vi "HFRR ADV v022 new software.vi"() -> ()   [LabVIEW 2025] (continued)
            n2951 = Match Pattern(string=w3831, regular expression=".dgf" ("substring (\"\")")) -> (before substring=w3841:string)  [unwired: 1 in, 3 out]
            n2952 = Concatenate Strings(w3841, ".duf" ("Substring")) -> (w3837:string)
            n2953 = String To Path(string=w3837) -> (path=w3842:path)
            n2954 = call <vilib>:"Read Characters From File.vi"("file path (dialog if empty)"=w3842, "start of read offset (chars.:0)"=60 ("start of read offset (chars.: 0)")) -> ("character string"=→"String Control 2":string)  [unwired: 4 in, 3 out]
          }
        }
        n2955 = case shown="True" "OPEN 2" {
          frame False {
          }
          frame True {
            (unwired) 0  # existing file
            w3863 = "Choose a datalog file to open"  # prompt
            n2956 = local write "OPEN 2"(FALSE ("OPEN 1")) -> ()
            n2957 = String To Path(string="C:\\LAB-IQ\\Data\\") -> (path=w3848:path)
            n2958 = File Dialog(6:"*.dgf" ("pattern"), 7:w3863, 11:w3848) -> (0:w3846:errorcluster, 3:w3854:path)  [unwired: 4 in, 2 out]
            n2959 = Unbundle(w3846) -> ()  [unwired: 3 out]
            n2960 = Strip Path(path=w3854) -> (name=w3852:string)  [unwired: 1 out]
            n2961 = Path To String(path=w3854) -> (string=w3849:string)
            "string1 2" <- w3849
            n2962 = Match Pattern(string=w3852, regular expression=".dgf") -> (before substring=→"String Control 3":string)  [unwired: 1 in, 3 out]
            n2963 = Match Pattern(string=w3849, regular expression=".dgf" ("substring (\"\")")) -> (before substring=w3860:string)  [unwired: 1 in, 3 out]
            n2964 = Concatenate Strings(w3860, ".duf" ("Substring")) -> (w3857:string)
            n2965 = String To Path(string=w3857) -> (path=w3855:path)
            n2966 = call <vilib>:"Read Characters From File.vi"("file path (dialog if empty)"=w3855, "start of read offset (chars.:0)"=60 ("start of read offset (chars.: 0)")) -> ("character string"=→"String Control 4":string)  [unwired: 4 in, 3 out]
          }
        }
        n2967 = case shown="True" "OPEN 3" {
          frame False {
          }
          frame True {
            (unwired) 0  # existing file
            w3881 = "Choose a datalog file to open"  # prompt
            n2968 = local write "OPEN 3"(FALSE ("OPEN 1")) -> ()
            n2969 = String To Path(string="C:\\LAB-IQ\\Data\\") -> (path=w3866:path)
            n2970 = File Dialog(6:"*.dgf" ("pattern"), 7:w3881, 11:w3866) -> (0:w3864:errorcluster, 3:w3872:path)  [unwired: 4 in, 2 out]
            n2971 = Unbundle(w3864) -> ()  [unwired: 3 out]
            n2972 = Strip Path(path=w3872) -> (name=w3870:string)  [unwired: 1 out]
            n2973 = Path To String(path=w3872) -> (string=w3867:string)
            "string1 3" <- w3867
            n2974 = Match Pattern(string=w3870, regular expression=".dgf") -> (before substring=→"String Control 5":string)  [unwired: 1 in, 3 out]
            n2975 = Match Pattern(string=w3867, regular expression=".dgf" ("substring (\"\")")) -> (before substring=w3877:string)  [unwired: 1 in, 3 out]
            n2976 = Concatenate Strings(w3877, ".duf" ("Substring")) -> (w3874:string)
            n2977 = String To Path(string=w3874) -> (path=w3878:path)
            n2978 = call <vilib>:"Read Characters From File.vi"("file path (dialog if empty)"=w3878, "start of read offset (chars.:0)"=60 ("start of read offset (chars.: 0)")) -> ("character string"=→"String Control 6":string)  [unwired: 4 in, 3 out]
          }
        }
        n2979 = case shown="True" "OPEN 4" {
          frame False {
          }
          frame True {
            (unwired) 0  # existing file
            w3899 = "Choose a datalog file to open"  # prompt
            n2980 = local write "OPEN 4"(FALSE ("OPEN 1")) -> ()
            n2981 = String To Path(string="C:\\LAB-IQ\\Data\\") -> (path=w3884:path)
            n2982 = File Dialog(6:"*.dgf" ("pattern"), 7:w3899, 11:w3884) -> (0:w3882:errorcluster, 3:w3890:path)  [unwired: 4 in, 2 out]
            n2983 = Unbundle(w3882) -> ()  [unwired: 3 out]
            n2984 = Strip Path(path=w3890) -> (name=w3888:string)  [unwired: 1 out]
            n2985 = Path To String(path=w3890) -> (string=w3885:string)
            "string1 4" <- w3885
            n2986 = Match Pattern(string=w3888, regular expression=".dgf") -> (before substring=→"String Control 7":string)  [unwired: 1 in, 3 out]
            n2987 = Match Pattern(string=w3885, regular expression=".dgf" ("substring (\"\")")) -> (before substring=w3895:string)  [unwired: 1 in, 3 out]
            n2988 = Concatenate Strings(w3895, ".duf" ("Substring")) -> (w3892:string)
            n2989 = String To Path(string=w3892) -> (path=w3896:path)
            n2990 = call <vilib>:"Read Characters From File.vi"("file path (dialog if empty)"=w3896, "start of read offset (chars.:0)"=60 ("start of read offset (chars.: 0)")) -> ("character string"=→"String Control 8":string)  [unwired: 4 in, 3 out]
          }
        }
      }
      frame "About" {
        # "Elapsed time\ncof\nstroke\nmean pos\nTemp\nHumidity"
        n2991 = disable-structure shown="Disabled" {
          frame Disabled {
            n2992 = case shown="True" "Export" {
              frame False {
              }
              frame True {
                w3921 = "                                      " ("string")
                w3923 = "\r"
                (unwired) i16 6 ("width (-)")
                w4000 = "\r"
                w3932 = "\r"
                n2993 = local write "Export"(FALSE ("Export")) -> ()
                n2994 = local read "String 29"() -> (w3969:string)
                n2995 = local read "String 34"() -> (w3957:string)
                n2996 = local read "String 35"() -> (w3952:string)
                n2997 = local read "String 37"() -> (w3948:string)
                n2998 = local read "String 36"() -> (w3945:string)
                n2999 = local read "String 38"() -> (w3942:string)
                n3000 = local read "String 39"() -> (w3939:string)
                n3001 = Match Pattern(string=w3969, regular expression=".dwm") -> (before substring=w3965:string)  [unwired: 1 in, 3 out]
                "before substring" <- w3965
                n3002 = local read "S 38"() -> (w3960:string)
                n3003 = local read "S 39"() -> (w3953:string)
                n3004 = local read "Temperature before test 2"() -> (w3989:dbl)
                n3005 = local read "Temperature after test 2"() -> (w3994:dbl)
                n3006 = local read "Humidity before test 2"() -> (w3975:dbl)
                n3007 = local read "Humidity after test 2"() -> (w3990:dbl)
                n3008 = local read "MWSD 2"() -> (w3986:dbl)
                n3009 = local read "WS1.4 2"() -> (w4002:dbl)
                n3010 = local read "HCF 2"() -> (w3998:dbl)
                n3011 = local read "AVP 2"() -> (w3987:dbl)
                n3012 = Concatenate Strings("1," ("string"), w3960) -> (w3959:string)
                n3013 = Concatenate Strings("2," ("string"), w3957) -> (w3956:string)
                n3014 = Concatenate Strings("3," ("string"), w3953) -> (w3955:string)
                n3015 = Concatenate Strings("4," ("string"), w3952) -> (w3951:string)
                n3016 = Concatenate Strings("5," ("string"), w3948) -> (w3949:string)
                n3017 = Concatenate Strings("6," ("string"), w3945) -> (w3946:string)
                n3018 = Concatenate Strings("7," ("string"), w3942) -> (w3943:string)
                n3019 = Concatenate Strings("8," ("string"), w3939) -> (w3940:string)
                n3020 = local read "Sample ID"() -> (w4007:string)
                n3021 = case shown="\"xlx\"" "Select File Type" {
                  tunnel: w3965 -> [w4010 w4012 w4014]
                  tunnel: [w4008 w4013 w4015] -> w3964
                  frame "xlx" {
                    n3022 = Concatenate Strings(w4010, ".xls" ("string")) -> (w4008:string)
                  }
                  frame "csv" {
                    n3023 = Concatenate Strings(w4012, ".csv" ("string")) -> (w4013:string)
                  }
                  frame "txt" {
                    n3024 = Concatenate Strings(w4014, ".txt" ("string")) -> (w4015:string)
                  }
                }
                n3025 = local read "Test Date"() -> (w4006:string)
                n3026 = local read "String 45"() -> (w3920:string)
                n3027 = local read "String 31"() -> (w4005:string)
                n3028 = local read "String 32"() -> (w4004:string)
                n3029 = local read "TITTLE"() -> (w3928:string)
                n3030 = Number To Fractional String(number=w3975, width (-)=i16 6, precision (6)=i16 2) -> (F-format string=w3974:string)  [unwired: 1 in]
                n3031 = Number To Fractional String(number=w3989, width (-)=i16 6, precision (6)=i16 2) -> (F-format string=w3995:string)  [unwired: 1 in]
                n3032 = Number To Fractional String(number=w3990, width (-)=i16 6, precision (6)=i16 2) -> (F-format string=w3988:string)  [unwired: 1 in]
                n3033 = Number To Fractional String(number=w3994, width (-)=i16 6, precision (6)=i16 2) -> (F-format string=w3993:string)  [unwired: 1 in]
                n3034 = Number To Fractional String(number=w3986, width (-)=i16 6, precision (6)=i16 2) -> (F-format string=w3984:string)  [unwired: 1 in]
                n3035 = Number To Fractional String(number=w3987, width (-)=i16 6, precision (6)=i16 2) -> (F-format string=w3985:string)  [unwired: 1 in]
                n3036 = Number To Fractional String(number=w3998, width (-)=i16 6, precision (6)=i16 2) -> (F-format string=w3999:string)  [unwired: 1 in]
                n3037 = Number To Fractional String(number=w4002, precision (6)=i16 2) -> (F-format string=w4003:string)  [unwired: 2 in]
                n3038 = local read "s.NO"() -> (w3922:string)
                n3039 = Concatenate Strings("=" ("string"), w3928) -> (w3927:string)
                n3040 = Concatenate Strings("S.No," ("string"), "                                       Parameters" ("string")) -> (w3933:string)
                n3041 = Concatenate Strings(w4000, w3959, w3974, w4000, w3956, w3995, w4000, w3955, w3988, w4000, w3951, w3993, w4000, w3949, w3984, w4000, w3946, w3985, w4000, w3943, w3999, w4000, w3940, w4003) -> (w3962:string)
                n3042 = Concatenate Strings(w3932, "," ("string"), w3920, w3922, w3921, w4004, w4007, w3921, w4005, w4006, w3932) -> (w3930:string)
                n3043 = local read "Tested by"() -> (w3936:string)
                n3044 = local read "String 33"() -> (w3937:string)
                n3045 = Concatenate Strings("," ("string"), "                                                                             " ("string")) -> (w3925:string)
                n3046 = Concatenate Strings(w3927, w3923, w3930, w3923, w3933, w3962, w3923, w3925, w3937, w3936) -> (→"export":string)
                n3047 = String To Path(string=w3964) -> (path=w3971:path)
                n3048 = local read "export"() -> (w3966:string)
                n3049 = call <vilib>:"Write Characters To File.vi"("append to file? (new file:F)"=FALSE, "character string"=w3966, "file path (dialog if empty)"=w3971) -> ()  [unwired: 2 in, 1 out]
              }
            }
          }
          frame Enabled {
          }
        }
        n3050 = case shown="True" "OK Button 17" {
          frame False {
          }
          frame True {
            (unwired) 0  # existing file
            w4224 = "Choose a datalog file to open"  # prompt
            n3051 = local write "OK Button 17"(FALSE ("OK Button 17")) -> ()
            n3052 = local read "String"() -> (w4219:string)
            n3053 = String To Path(string=w4219) -> (path=w4220:path)
            n3054 = File Dialog(6:"*.duf" ("pattern"), 7:w4224, 11:w4220) -> (0:w4211:errorcluster, 3:w4230:path)  [unwired: 4 in, 2 out]
            n3055 = Unbundle(w4211) -> ()  [unwired: 3 out]
            n3056 = Open/Create/Replace File "Open File"(file path (use dialog)=w4230) -> (refnum out=w4222:refnum<file>)  [unwired: 5 in, 2 out]
            n3057 = Strip Path(path=w4230) -> (name=w4228:string)  [unwired: 1 out]
            n3058 = Path To String(path=w4230) -> (string=w4213:string)
            n3059 = while {
              tunnel: w4222 -> [w4234]
              i -> [w4231]
              stop <- w4232 continue-if-true
              (unwired) TRUE ("line mode (F)")
              n3060 = Read from Text File "Read File"(file (use dialog)=w4234) -> (text=w4233:string)  [unwired: 3 in, 3 out]
              n3061 = local write "Numeric 16"(w4231) -> ()
              n3062 = String Length(string=w4233) -> (length=w4236:i32)
              n3063 = Greater?(x=w4236, y=1) -> (0:w4232:bool)
            }
            n3064 = local write "String 29"(w4213) -> ()
            n3065 = Search and Replace String(input string=w4213, search string=".duf", replace string=".dgf" ("replace string (\"\")")) -> (result string=→"String Indicator 4":string)  [unwired: 5 in, 3 out]
            n3066 = Match Pattern(string=w4228, regular expression=".dwm") -> (before substring=w4212:string)  [unwired: 1 in, 3 out]
            "String Indicator" <- w4212
            n3067 = Match Pattern(string=w4213, regular expression=".dwm" ("substring (\"\")")) -> (before substring=w4214:string)  [unwired: 1 in, 3 out]
            "String Indicator 3" <- w4214
            n3068 = local write "TITTLE 2"(w4212) -> ()
            n3069 = String To Path(string=w4214) -> (path=w4221:path)
            "path" <- w4221
            n3070 = call <vilib>:"Read Characters From File.vi"("file path (dialog if empty)"=w4221, "start of read offset (chars.:0)"=60 ("start of read offset (chars.: 0)")) -> ("character string"=→"String Indicator 2":string)  [unwired: 4 in, 3 out]
          }
        }
        n3071 = call <vilib>:"Query Available Printers.vi"() -> ("system configured printers"=w3913:string[])  [unwired: 9 in, 2 out]
        "System Configured Printers 2" <- w3913
        n3072 = local read "OK Button 16"() -> (w3910:bool)
        n3073 = case shown="True" "OK Button 16" {
          frame False {
          }
          frame True {
            n3074 = stacked-sequence {
              frame #0 {
                n3075 = local read "Numeric 16"() -> (w4238:i32)
                n3076 = local write "Numeric 10"(w4238) -> ()
              }
              frame #1 {
                n3077 = local read "S.NO"() -> (→"s.NO":string)
                n3078 = local read "String 29"() -> (w4242:string)
                n3079 = String To Path(string=w4242) -> (path=w4241:path)
                n3080 = Open/Create/Replace File "Open File"(file path (use dialog)=w4241) -> (refnum out=w4243:refnum<file>)  [unwired: 5 in, 2 out]
                n3081 = for {
                  N: 16 -> [_]
                  tunnel: w4243 -> [w4250]
                  i -> [w4246]
                  (unwired) TRUE ("line mode (F)")
                  n3082 = Read from Text File "Read File"(file (use dialog)=w4250) -> (text=w4244:string)  [unwired: 3 in, 3 out]
                  n3083 = Match Pattern(string=w4244, regular expression="(") -> (after substring=w4249:string)  [unwired: 1 in, 3 out]
                  n3084 = Match Pattern(string=w4249, regular expression=")") -> (before substring=w4245:string)  [unwired: 1 in, 3 out]
                  n3085 = case shown="1" w4246 {
                    tunnel: w4245 -> [w4251 w4252 _ _ w4253 w4254 w4255 w4257 w4259 w4261 w4263 w4265 w4267 w4269 _]
                    tunnel: w4244 -> [_ _ _ _ _ _ _ _ _ _ _ _ _ _ _]
                    frame 0 {
                      "TITTLE" <- w4251
                    }
                    frame 1 {
                      "Sample ID" <- w4252
                    }
                    frame 2 {
                    }
                    frame 3 {
                    }
                    frame 4 {
                      "Test Date" <- w4253
                    }
                    frame 5 {
                      "Tested by" <- w4254
                    }
                    frame 6 {
                      n3086 = Fract/Exp String To Number(string=w4255) -> (number=→"Humidity before test 2":dbl)  [unwired: 3 in, 1 out]
                    }
                    frame 7 {
                      n3087 = Fract/Exp String To Number(string=w4257) -> (number=→"Temperature before test 2":dbl)  [unwired: 3 in, 1 out]
                    }
                    frame 8 {
                      n3088 = Fract/Exp String To Number(string=w4259) -> (number=→"Humidity after test 2":dbl)  [unwired: 3 in, 1 out]
                    }
                    frame 9 {
                      n3089 = Fract/Exp String To Number(string=w4261) -> (number=→"Temperature after test 2":dbl)  [unwired: 3 in, 1 out]
                    }
                    frame 10 {
                      n3090 = Fract/Exp String To Number(string=w4263) -> (number=→"MWSD 2":dbl)  [unwired: 3 in, 1 out]
                    }
                    frame 11 {
                      n3091 = Fract/Exp String To Number(string=w4265) -> (number=→"AVP 2":dbl)  [unwired: 3 in, 1 out]
                    }
                    frame 12 {
                      n3092 = Fract/Exp String To Number(string=w4267) -> (number=→"HCF 2":dbl)  [unwired: 3 in, 1 out]
                    }
                    frame 13 {
                      n3093 = Fract/Exp String To Number(string=w4269) -> (number=→"WS1.4 2":dbl)  [unwired: 3 in, 1 out]
                    }
                    frame 14, Default {
                    }
                  }
                }
              }
              frame #2 {
              }
            }
            n3094 = local write "OK Button 16"(FALSE ("OK Button 13")) -> ()
          }
        }
        n3095 = Index Array(array=w3913, index="Select Printer 3") -> (element=w3915:string)
        "Selected Printer" <- w3915
        n3096 = case shown="True" w3910 {
          frame False {
          }
          frame True {
            n3097 = flat-sequence {
              frame #0 {
              }
              frame #1 {
                n3098 = Wait (ms)(milliseconds to wait=u32 100) -> ()  [unwired: 1 out]
              }
              frame #2 {
                n3099 = local write "OK Button 16"(FALSE ("Print 3")) -> ()
              }
            }
          }
        }
        n3100 = case shown="True" "Print" {
          tunnel: w3915 -> [_ w4207]
          frame False {
          }
          frame True {
            (unwired) i16 6 ("width (-)")
            (unwired) "TESTED BY : "
            (unwired) "TESTED DATE :"
            (unwired) "SAMPLE ID : "
            (unwired) "SAMPLE DESIGN : "
            w4165 = "\r"
            w4182 = "\r"
            # "add image"
            n3101 = local read "Sample ID"() -> (w4155:string)
            n3102 = local read "Tested by"() -> (w4158:string)
            n3103 = local read "String 34"() -> (w4145:string)
            n3104 = local read "String 45"() -> (w4125:string)
            n3105 = local read "String 35"() -> (w4140:string)
            n3106 = local read "String 37"() -> (w4138:string)
            n3107 = local read "String 32"() -> (w4160:string)
            n3108 = local read "String 36"() -> (w4135:string)
            n3109 = local read "String 31"() -> (w4159:string)
            n3110 = local read "Test Date"() -> (w4156:string)
            n3111 = local read "String 33"() -> (w4161:string)
            n3112 = local read "String 38"() -> (w4131:string)
            n3113 = local read "String 39"() -> (w4128:string)
            n3114 = local write "Print"(FALSE ("Print FF")) -> ()
            n3115 = local read "S 39"() -> (w4143:string)
            n3116 = local read "S 38"() -> (w4150:string)
            n3117 = local read "Temperature before test 2"() -> (w4181:dbl)
            n3118 = local read "Temperature after test 2"() -> (w4171:dbl)
            n3119 = local read "Humidity before test 2"() -> (w4196:dbl)
            n3120 = local read "Humidity after test 2"() -> (w4180:dbl)
            n3121 = local read "MWSD 2"() -> (w4185:dbl)
            n3122 = local read "WS1.4 2"() -> (w4163:dbl)
            n3123 = Concatenate Strings("2)" ("string"), w4145) -> (w4146:string)
            n3124 = Concatenate Strings("3)" ("string"), w4143) -> (w4144:string)
            n3125 = Concatenate Strings("1)" ("string"), w4150) -> (w4149:string)
            n3126 = Concatenate Strings("4)" ("string"), w4140) -> (w4141:string)
            n3127 = Concatenate Strings("5)" ("string"), w4138) -> (w4137:string)
            n3128 = Concatenate Strings("6)" ("string"), w4135) -> (w4134:string)
            n3129 = Concatenate Strings("7)" ("string"), w4131) -> (w4132:string)
            n3130 = Concatenate Strings("8)" ("string"), w4128) -> (w4129:string)
            n3131 = local read "HCF 2"() -> (w4167:dbl)
            n3132 = local read "AVP 2"() -> (w4184:dbl)
            n3133 = local read "s.NO"() -> (w4126:string)
            n3134 = call <vilib>:"New Report.vi"("report type"=enum16{"Standard Report", "HTML"}."Standard Report") -> ("report out"=w4205:refnum<class "NI_report.lvclass">, "error out"=w4204:errorcluster)  [unwired: 13 in]
            n3135 = local read "TITTLE"() -> (w4157:string)
            n3136 = Concatenate Strings(w4182, w4125, w4126, w4182, w4160, w4155, w4182, w4159, w4156, w4182, w4161, w4158, w4182) -> (w4175:string)
            "test by" <- w4175
            n3137 = Number To Fractional String(number=w4181, width (-)=i16 6, precision (6)=i16 2) -> (F-format string=w4170:string)  [unwired: 1 in]
            n3138 = Number To Fractional String(number=w4180, width (-)=i16 6, precision (6)=i16 2) -> (F-format string=w4183:string)  [unwired: 1 in]
            n3139 = Number To Fractional String(number=w4196, width (-)=i16 6, precision (6)=i16 2) -> (F-format string=w4201:string)  [unwired: 1 in]
            n3140 = Number To Fractional String(number=w4185, width (-)=i16 6, precision (6)=i16 2) -> (F-format string=w4187:string)  [unwired: 1 in]
            n3141 = Number To Fractional String(number=w4171, width (-)=i16 6, precision (6)=i16 2) -> (F-format string=w4172:string)  [unwired: 1 in]
            n3142 = Number To Fractional String(number=w4184, width (-)=i16 6, precision (6)=i16 2) -> (F-format string=w4186:string)  [unwired: 1 in]
            n3143 = Number To Fractional String(number=w4167, width (-)=i16 6, precision (6)=i16 2) -> (F-format string=w4166:string)  [unwired: 1 in]
            n3144 = Number To Fractional String(number=w4163, precision (6)=i16 2) -> (F-format string=w4162:string)  [unwired: 2 in]
            n3145 = call-dynamic "Set Report Header Text.vi"("report in"=w4205, "center header text"=w4157, "error in (no error)"=w4204) -> ("report out"=w4176:refnum<class "NI_report.lvclass">, "error out"=w4177:errorcluster)  [unwired: 11 in]
            n3146 = Concatenate Strings(w4165, w4149, w4201, w4165, w4146, w4170, w4165, w4144, w4183, w4165, w4141, w4172, w4165, w4137, w4187, w4165, w4134, w4186, w4165, w4132, w4166, w4165, w4129, w4162) -> (w4153:string)
            "export 2" <- w4153
            n3147 = call-poly <vilib>:"Append Report Text.vi"("report in"=w4176, "text"=w4175, "error in (no error)"=w4177) -> ("report out"=w4179:refnum<class "NI_report.lvclass">, "error out"=w4178:errorcluster)  [unwired: 9 in, 2 out]
            n3148 = local read "test by"() -> (w4152:string)
            n3149 = local read "TITTLE"() -> (w4154:string)
            n3150 = call-poly <vilib>:"Append Report Text.vi"("report in"=w4179, "error in (no error)"=w4178) -> ("report out"=w4200:refnum<class "NI_report.lvclass">, "error out"=w4198:errorcluster)  [unwired: 10 in, 2 out]
            n3151 = Concatenate Strings(w4154, w4153, w4152) -> (→"output":string)
            n3152 = call-poly <vilib>:"Append Report Text.vi"("report in"=w4200, "text"=w4153, "error in (no error)"=w4198) -> ("report out"=w4199:refnum<class "NI_report.lvclass">, "error out"=w4197:errorcluster)  [unwired: 9 in, 2 out]
            n3153 = call-dynamic "Print Report.vi"("report in"=w4199, "printer name (default)"=w4207, "error in (no error)"=w4197) -> ("report out"=w4209:refnum<class "NI_report.lvclass">, "error out"=w4210:errorcluster)  [unwired: 11 in]
            n3154 = call-dynamic "Dispose Report.vi"("report in"=w4209, "error in (no error)"=w4210) -> ()  [unwired: 13 in, 1 out]
          }
        }
        n3155 = case shown="True" "Print 2" {
          frame False {
          }
          frame True {
            n3156 = flat-sequence {
              frame #0 {
                n3157 = local read "s.NO"() -> (→"s.NO 2":string)
                n3158 = Wait (ms)(milliseconds to wait=u32 20) -> ()  [unwired: 1 out]
                n3159 = local read "Sample ID  3"() -> (→"Sample ID  6":string)
                n3160 = local read "Sample ID  4"() -> (→"Sample ID  7":string)
                n3161 = local read "Sample ID"() -> (→"Sample ID  2":string)
                n3162 = local read "Tested by"() -> (→"Tested by 2":string)
                n3163 = local read "Test Date"() -> (→"Test Date 2":string)
                n3164 = local read "Humidity after test 3"() -> (→"Humidity after test 4":dbl)
                n3165 = local read "Ref A Test Date :"() -> (→"TITTLE 4":string)
                n3166 = local read "Temperature before test 3"() -> (w4032:dbl)
                n3167 = local read "Temperature before test 3"() -> (→"Temperature after test 5":dbl)
                n3168 = local read "Temperature after test 3"() -> (→"Temperature after test 4":dbl)
                n3169 = local read "Humidity before test 3"() -> (→"Humidity before test 4":dbl)
                n3170 = local write "Temperature before test 3"(w4032) -> ()
                n3171 = local read "image data"() -> (w4023:T16)
                n3172 = String To Path(string="C:\\LAB-IQ\\im\\Temp_resized.jpg") -> (path=w4024:path)
                "path 2" <- w4024
                n3173 = call <vilib>:"Write JPEG File.vi"("image data"=w4023, "path to JPEG file"=w4024) -> ()  [unwired: 8 in, 2 out]
                "Ref A Test Date :" <- "Ref A Test Date :"
                "Ref B Test Date :" <- "Ref B Test Date :"
                "Ref B Scar Value :" <- "Ref B Scar Value :"
                "Ref A Scar Value :" <- "Ref A Scar Value :"
              }
              frame #1 {
                (unwired) HTML_Report_Image_Alignment."MIDDLE" ("alignment (default)")
                w4060 = u16 0 items=["portrait", "landscape"] ("orientation (portrait)")
                (unwired) HTML_Report_Image_Alignment."ABSMIDDLE" ("alignment (default)")
                (unwired) "TESTED BY : "
                (unwired) "TESTED DATE :"
                (unwired) "SAMPLE ID : "
                (unwired) "SAMPLE DESIGN : "
                w4093 = "\r"
                # "add image"
                n3174 = Wait (ms)(milliseconds to wait=u32 20) -> ()  [unwired: 1 out]
                n3175 = local read "Sample ID  2"() -> (w4086:string)
                n3176 = local read "Wear Scar X"() -> (w4058:dbl)
                "Length ( microns ) 2" <- w4058
                n3177 = local read "Wear Scar Y"() -> (w4057:dbl)
                "Wear Scar Y ( microns ) :" <- w4057
                n3178 = local read "Test Date 2"() -> (w4087:string)
                n3179 = local read "Tested by 2"() -> (w4088:string)
                n3180 = local read "String 46"() -> (w4084:string)
                n3181 = local read "String 48"() -> (w4090:string)
                n3182 = local read "String 47"() -> (w4089:string)
                n3183 = local read "String 49"() -> (w4091:string)
                n3184 = local read "String 10"() -> (w4044:string)
                n3185 = local read "s.NO 2"() -> (w4085:string)
                n3186 = Add(x=w4058, y=w4057) -> (x+y=w4056:dbl)
                n3187 = call <vilib>:"New Report.vi"("report type"=enum16{"Standard Report", "HTML"}."HTML") -> ("report out"=w4064:refnum<class "NI_report.lvclass">, "error out"=w4062:errorcluster)  [unwired: 13 in]
                n3188 = Concatenate Strings(w4093, w4084, w4085, w4093, w4090, w4086, w4093, w4089, w4087, w4093, w4091, w4088, w4093) -> (→"test by 2":string)
                n3189 = Concatenate Strings("C:\\LAB-IQ\\Data\\" ("string"), w4044, ".jpg" ("string")) -> ()  [unwired: 1 out]
                n3190 = Divide(x=w4056, y=2.0) -> (x/y=→"Mean Wear ( microns) :":dbl)
                n3191 = call-dynamic "Set Report Orientation.vi"("report in"=w4064, "orientation (portrait)"=w4060, "error in (no error)"=w4062) -> ("report out"=w4063:refnum<class "NI_report.lvclass">, "error out"=w4061:errorcluster)  [unwired: 11 in]
                n3192 = for {
                  N: 5 -> [_]
                  tunnel: w4063 -> [w4114]
                  tunnel: [w4113] -> w4042
                  tunnel: w4061 -> [w4112]
                  tunnel: [w4111] -> w4041
                  n3193 = call-dynamic "Set Report Tab Width.vi"("report in"=w4114, "error in (no error)"=w4112) -> ("report out"=w4113:refnum<class "NI_report.lvclass">, "error out"=w4111:errorcluster)  [unwired: 12 in]
                }
                n3194 = local read "TITTLE"() -> (w4059:string)
                n3195 = call-dynamic "Set Report Header Text.vi"("report in"=w4042, "center header text"=w4059, "error in (no error)"=w4041) -> ("report out"=w4080:refnum<class "NI_report.lvclass">, "error out"=w4079:errorcluster)  [unwired: 11 in]
                n3196 = for {
                  N: 1 -> [_]
                  tunnel: [w4118] -> w4066
                  tunnel: [w4117] -> w4065
                  tunnel: w4080 -> [w4116]
                  tunnel: w4079 -> [w4115]
                  n3197 = call-dynamic "New Report Line.vi"("report in"=w4116, "error in (no error)"=w4115) -> ("report out"=w4118:refnum<class "NI_report.lvclass">, "error out"=w4117:errorcluster)  [unwired: 12 in]
                }
                n3198 = for {
                  N: 2 -> [_]
                  tunnel: [w4110] -> w4072
                  tunnel: [w4109] -> w4071
                  tunnel: w4066 -> [w4108]
                  tunnel: w4065 -> [w4107]
                  n3199 = call-dynamic "New Report Line.vi"("report in"=w4108, "error in (no error)"=w4107) -> ("report out"=w4110:refnum<class "NI_report.lvclass">, "error out"=w4109:errorcluster)  [unwired: 12 in]
                }
                n3200 = for {
                  N: 25 -> [_]
                  tunnel: w4072 -> [w4106]
                  tunnel: w4071 -> [w4104]
                  tunnel: [w4105] -> w4075
                  tunnel: [w4103] -> w4074
                  n3201 = call-dynamic "Set Report Tab Width.vi"("report in"=w4106, "error in (no error)"=w4104) -> ("report out"=w4105:refnum<class "NI_report.lvclass">, "error out"=w4103:errorcluster)  [unwired: 12 in]
                }
                n3202 = control-ref of="Tab Control 9"() -> (w4070:refnum<vi>)
                n3203 = call-dynamic "Append Control Image to Report.vi"("report in"=w4075, "alignment (default)"=HTML_Report_Image_Alignment."ABSMIDDLE", "ctrl reference"=w4070, "error in (no error)"=w4074) -> ("report out"=w4069:refnum<class "NI_report.lvclass">, "error out"=w4068:errorcluster)  [unwired: 8 in, 2 out]
                n3204 = for {
                  N: 3 -> [_]
                  tunnel: [w4102] -> w4053
                  tunnel: [w4101] -> w4052
                  tunnel: w4069 -> [w4100]
                  tunnel: w4068 -> [w4099]
                  n3205 = call-dynamic "New Report Line.vi"("report in"=w4100, "error in (no error)"=w4099) -> ("report out"=w4102:refnum<class "NI_report.lvclass">, "error out"=w4101:errorcluster)  [unwired: 12 in]
                }
                n3206 = for {
                  N: 100 -> [_]
                  tunnel: w4053 -> [w4098]
                  tunnel: w4052 -> [w4096]
                  tunnel: [w4097] -> w4049
                  tunnel: [w4095] -> w4047
                  n3207 = call-dynamic "Set Report Tab Width.vi"("report in"=w4098, "error in (no error)"=w4096) -> ("report out"=w4097:refnum<class "NI_report.lvclass">, "error out"=w4095:errorcluster)  [unwired: 12 in]
                }
                n3208 = String To Path(string="C:\\LAB-IQ\\im\\Temp_resized.jpg") -> (path=w4039:path)
                n3209 = call-poly <vilib>:"Append Image to Report.vi"("report in"=w4049, "path or URL of image"=w4039, "error in (no error)"=w4047) -> ("report out"=w4048:refnum<class "NI_report.lvclass">, "error out"=w4046:errorcluster)  [unwired: 9 in, 2 out]
                n3210 = call-poly <vilib>:"Open HTML Report in Browser.vi"("report in"=w4048, "error in (no error)"=w4046) -> ("report out"=w4083:refnum<class "NI_report.lvclass">, "error out"=w4082:errorcluster)  [unwired: 11 in, 1 out]
                n3211 = call-dynamic "Dispose Report.vi"("report in"=w4083, "error in (no error)"=w4082) -> ()  [unwired: 13 in, 1 out]
              }
              frame #2 {
              }
              frame #3 {
                n3212 = disable-structure shown="Disabled" {
                  frame Disabled {
                    n3213 = local read "String 10"() -> (w4123:string)
                    n3214 = Concatenate Strings("C:\\LAB-IQ-NXT\\Data\\" ("string"), w4123, ".jpg" ("string")) -> (w4121:string)
                    n3215 = String To Path(string=w4121) -> (path=w4120:path)
                    n3216 = Delete(path (use dialog)=w4120) -> ()  [unwired: 4 in, 3 out]
                  }
                  frame Enabled {
                  }
                }
                n3217 = local write "Print 2"(FALSE ("Print")) -> ()
              }
            }
          }
        }
      }
    }
    n3218 = property on="SetTemp" class="DigNum (strict)"("Disabled"=w2059) -> ()  [unwired: 2 in, 2 out]
    n3219 = Multiply(x=w2049, y=w2051) -> (x*y=w2050:dbl)
    n3220 = local read "MWSD"() -> (w2048:dbl)
    n3221 = Add(x=w2050, y=w2048) -> (x+y=→"WS1.4":dbl)
    n3222 = Wait (ms)(milliseconds to wait=u32 50) -> ()  [unwired: 1 out]
    n3223 = Wait (ms)(milliseconds to wait=u32 50) -> ()  [unwired: 1 out]
    n3224 = local read "Quit"() -> (w2047:bool)
  }
  n3225 = VISA Close(VISA resource name=w43, error in (no error)=w42) -> ()  [unwired: 1 out]
  n3226 = while {
    tunnel: [w4284] -> w52
    shift-right: [w4277] -> _
    shift-left: 0.0 -> [w4280]
    shift-right: [w4276] -> _
    shift-left: 0.0 -> [w4279]
    shift-right: [w4275] -> _
    shift-left: 100.0 ("vc_cmd") -> [w4278]
    stop <- w4284 stop-if-true
    # "PID LOGIC"
    n3227 = local read "RUN"() -> (w4282:bool)
    n3228 = local read "Auto Start Temp"() -> (w4271:bool)
    n3229 = local read "Auto Start Test"() -> (w4281:bool)
    n3230 = local read "START TEMP"() -> (w4273:bool)
    n3231 = And(x=w4271, y=w4281) -> (x .and. y?=w4272:bool)
    n3232 = Or(x=w4282, y=w4272) -> (x .or. y?=w4283:bool)
    n3233 = And(x=w4283, y=w4273) -> (x .and. y?=w4274:bool)
    n3234 = Wait (ms)(milliseconds to wait=u32 20) -> ()  [unwired: 1 out]
    n3235 = case shown="True" w4274 {
      tunnel: [400.0 ("out_vc_cmd") w4304] -> w4275
      tunnel: [w4287 w4306] -> w4276
      tunnel: [w4287 w4305] -> w4277
      tunnel: w4280 -> [_ w4295]
      tunnel: w4279 -> [_ w4294]
      tunnel: w4278 -> [_ w4293]
      frame False {
        w4287 = 0.0 ("error_out")
      }
      frame True {
        n3236 = local read "Set Strk"() -> (w4290:dbl)
        n3237 = local read "LVDT STROKE"() -> (w4288:dbl)
        n3238 = Add(x=w4290, y="Add up Stroke") -> (x+y=w4291:dbl)
        n3239 = formula code="// Zero-Hardcode Explicit Positional-Form PID Engine\n// Inputs: target_stroke, measured_stroke, dt, prev_error, integral_accumulator_in, prev_vc_cmd\n//         kp, ki, kd, max_step_change, max_amplitude, min_amplitude, startup_cmd\n// Outputs: vc_cmd, error_out, out_error, integral_accumulator_out, out_vc_cmd\n\n// 1. Calculate Tracking Error\nfloat current_error = target_stroke - measured_stroke;\nerror_out = current_error;\n\n// 2. Compute Proportional Term\nfloat p_term = kp * current_error;\n\n// 3. Compute Derivative Term\nfloat d_term = 0.0;\nif (dt > 0.0) {\n    d_term = kd * ((current_error - prev_error) / dt);\n}\n\n// 4. Update and Accumulate Integral Term\nfloat current_integral = integral_accumulator_in + (current_error * dt);\nfloat i_term = ki * current_integral;\n\n// 5. Calculate Ideal Target Command\nfloat ideal_command = startup_cmd + p_term + i_term + d_term;\n\n// 6. Anti-Windup Protection (Back-calculation method)\nif (ideal_command > max_amplitude) {\n    float excess = ideal_command - max_amplitude;\n    if (ki > 0.0) {\n        current_integral -= excess / ki;\n    }\n    ideal_command = max_amplitude;\n} else if (ideal_command < min_amplitude) {\n    float excess = ideal_command - min_amplitude;\n    if (ki > 0.0) {\n        current_integral -= excess / ki;\n    }\n    ideal_command = min_amplitude;\n}\n\n// 7. Apply Loop Rate Limiting (Protects voice coil from large voltage steps)\nfloat raw_adjustment = ideal_command - prev_vc_cmd;\n\nif (raw_adjustment > max_step_change) {\n    raw_adjustment = max_step_change;\n} else if (raw_adjustment < -max_step_change) {\n    raw_adjustment = -max_step_change;\n}\n\nfloat next_vc_cmd = prev_vc_cmd + raw_adjustment;\n\n// Final Output Safety Safeguard Clamping\nif (next_vc_cmd > max_amplitude) {\n    next_vc_cmd = max_amplitude;\n} else if (next_vc_cmd < min_amplitude) {\n    next_vc_cmd = min_amplitude;\n}\n\n// 8. Map to Shift Registers for memory persistence\nvc_cmd = next_vc_cmd;\nout_error = current_error;                     \nintegral_accumulator_out = current_integral;  \nout_vc_cmd = next_vc_cmd;"("target_stroke"=w4291, "measured_stroke"=w4288, "dt"="dt", "integral_accumulator_in"=w4294, "prev_error"=w4295, "prev_vc_cmd"=w4293, "kp"="kp", "ki"="ki", "kd"="kd", "max_step_change"="max_step_change", "max_amplitude"="max_amplitude", "min_amplitude"="min_amplitude", "startup_cmd"="startup_cmd") -> ("vc_cmd"=w4310:dbl, "out_error"=w4305:dbl, "integral_accumulator_out"=w4306:dbl, "out_vc_cmd"=w4304:dbl)  [unwired: 1 out]
        "output Vpp" <- w4310
        n3240 = Number To Fractional String(number=w4310, precision (6)=i16 1) -> (F-format string=w4308:string)  [unwired: 2 in]
        n3241 = Concatenate Strings("DAC;" ("string"), w4308) -> (w4292:string)
        n3242 = local write "Command"(w4292) -> ()
        "prev_error" <- w4295
        "integral_accumulator_in" <- w4294
        "prev_vc_cmd" <- w4293
      }
    }
    n3243 = local read "Quit"() -> (w4284:bool)
  }
  n3244 = Or(x=w48, y=w47) -> (x .or. y?=w49:bool)
  n3245 = Or(x=w45, y=w49) -> (x .or. y?=w54:bool)
  n3246 = control-ref of="new picture"() -> ()  [unwired: 1 out]
  n3247 = Or(x=w57, y=w54) -> (x .or. y?=w51:bool)
  n3248 = Or(x=w51, y=w52) -> (x .or. y?=w46:bool)
  n3249 = while {
    tunnel: [w4311] -> w56
    i -> [w4318]
    stop <- w4311 stop-if-true
    n3250 = local read "Quit"() -> (w4311:bool)
    n3251 = Equal To 0?(x=w4318) -> (x = 0?=w4316:bool)
    n3252 = call "Elapsed Time3"("Time Target (s)"=45.0, "Auto Reset"=TRUE) -> ("Time has Elapsed"=w4315:bool)  [unwired: 10 in, 7 out]
    n3253 = Wait (ms)(milliseconds to wait=u32 50) -> ()  [unwired: 1 out]
    n3254 = Or(x=w4315, y=w4316) -> (x .or. y?=w4317:bool)
    n3255 = case shown="True" w4317 {
      frame False {
      }
      frame True {
        n3256 = call <vilib>:"System Exec.vi"("run minimized? (F)"=TRUE, "error in (no error)"="error in (no error)", "command line"="powercfg.exe -change -monitor-timeout-ac 0") -> ("error out"=w4329:errorcluster)  [unwired: 5 in, 3 out]
        n3257 = call <vilib>:"System Exec.vi"("run minimized? (F)"=TRUE, "error in (no error)"=w4329, "command line"="powercfg.exe -change -disk-timeout-ac 0") -> ("error out"=w4328:errorcluster)  [unwired: 5 in, 3 out]
        n3258 = call <vilib>:"System Exec.vi"("run minimized? (F)"=TRUE, "error in (no error)"=w4328, "command line"="powercfg.exe -change -standby-timeout-ac 0") -> ("error out"=w4327:errorcluster)  [unwired: 5 in, 3 out]
        n3259 = call <vilib>:"System Exec.vi"("run minimized? (F)"=TRUE, "error in (no error)"=w4327, "command line"="powercfg.exe -change -hibernate-timeout-ac 0") -> ("error out"=w4326:errorcluster)  [unwired: 5 in, 3 out]
        n3260 = call <vilib>:"Simple Error Handler.vi"("error in (no error)"=w4326) -> ("error out"=w4332:errorcluster)  [unwired: 4 in, 4 out]
        n3261 = call <vilib>:"Clear Errors.vi"("error in (no error)"=w4332) -> ("error out"=→"error out":errorcluster)  [unwired: 5 in, 1 out]
      }
    }
  }
  n3262 = Compound Arithmetic op=OR(w59, w46, w56) -> (w58:bool)
  n3263 = flat-sequence {
    tunnel: w58 -> [_]
    tunnel: [w4334] -> w24
    tunnel: w24 -> [_]
    frame #0 {
      n3264 = call "CLOSE CONNECTION.vi"() -> ("error out"=w4334:errorcluster)  [unwired: 11 in]
    }
    frame #1 {
      n3265 = Quit LabVIEW(quit? (T)=TRUE) -> ()
      n3266 = local write "Quit"(FALSE ("EXIT")) -> ()
    }
  }
  n3267 = property on="Heater Button" class="Bool (strict)"("Visible"=TRUE) -> ()  [unwired: 2 in, 2 out]
  n3268 = disable-structure shown="Disabled" {
    disable-tunnel: _ -> [w4340 _]
    disable-tunnel: _ -> [w4337 _]
    disable-tunnel: _ -> [w4338 _]
    frame Disabled {
      n3269 = disable-structure shown="Disabled" {
        disable-tunnel: [w4347 _] -> w4339
        frame Disabled {
          n3270 = while {
            shift-right: [w4389] -> w4345
            shift-left: errorcluster {"status"=TRUE, "code"=0, "source"="Init"} ("error out") -> [w4354]
            shift-right: [w4388] -> w4344
            shift-left: _ -> [w4355]
            shift-right: [w4387] -> _
            shift-left: "" -> [w4386]
            tunnel: [w4348] -> w4347
            shift-right: ["Set Rh"] -> _
            shift-left: 0.0 ("Set Rh") -> [w4380]
            tunnel: [w4357] -> _
            i -> [w4357]
            stop <- w4348 stop-if-true
            n3271 = flat-sequence {
              tunnel: w4354 -> [w4392]
              tunnel: [w4392] -> w4353
              frame #0 {
                n3272 = Wait (ms)(milliseconds to wait=u32 200) -> ()  [unwired: 1 out]
              }
            }
            n3273 = local read "Com Port 3"() -> (w4356:refnum<visa-resource-name>)
            n3274 = local read "Humidity Str Rec"() -> (w4358:string)
            n3275 = Not Equal?(x="Set Rh", y=w4380) -> (x != y?=w4385:bool)
            n3276 = Number To Decimal String(number="Set Rh") -> (decimal integer string=w4383:string)  [unwired: 1 in]
            n3277 = Not Equal?(x=w4356, y=w4355) -> (x != y?=w4351:bool)
            n3278 = Concatenate Strings("#setPoint00" ("string"), w4383) -> (w4384:string)
            n3279 = case shown="False" w4385 {
              tunnel: w4384 -> [_ w4404]
              frame False {
                n3280 = local read "Humidity"() -> (w4401:bool)
                n3281 = case shown="True" w4401 {
                  frame False {
                    n3282 = local write "Humidity Str Send"("stop" ("Humidity Str Send")) -> ()
                  }
                  frame True {
                    n3283 = local write "Humidity Str Send"("start" ("Humidity Str Send")) -> ()
                  }
                }
              }
              frame True {
                n3284 = local write "Humidity Str Send"(w4404) -> ()
              }
            }
            n3285 = Or(x=w4351) -> (y=w4349:bool, x .or. y?=w4350:bool)
            n3286 = String Subset(string=w4358, offset (0)=7) -> (substring=w4373:string)  [unwired: 1 in]
            n3287 = Match Pattern(string=w4358, regular expression="?") -> (offset past match=w4376:i32)  [unwired: 1 in, 3 out]
            n3288 = Match Pattern(string=w4358, regular expression="v") -> (offset past match=w4379:i32)  [unwired: 1 in, 3 out]
            n3289 = case shown="True" w4350 {
              tunnel: w4353 -> [w4390 _]
              tunnel: [w4390 errorcluster {"status"=TRUE, "code"=0, "source"="Init"} ("error out")] -> w4352
              frame False {
              }
              frame True {
              }
            }
            n3290 = Equal?(x=w4376, y=-1) -> (x = y?=w4360:bool)
            n3291 = Match Pattern(string=w4373, regular expression="g") -> (after substring=w4374:string, offset past match=w4365:i32)  [unwired: 1 in, 2 out]
            n3292 = Match Pattern(string=w4373, regular expression="y") -> (after substring=w4372:string, offset past match=w4366:i32)  [unwired: 1 in, 2 out]
            n3293 = Greater?(x=w4366, y=w4365) -> (0:w4371:bool)
            n3294 = Greater Or Equal To 0?(x=w4366) -> (x >= 0?=w4363:bool)
            n3295 = Greater Or Equal To 0?(x=w4365) -> (x >= 0?=w4364:bool)
            n3296 = Or(x=w4363, y=w4364) -> (x .or. y?=w4362:bool)
            n3297 = Greater Or Equal To 0?(x=w4379) -> (x >= 0?=w4361:bool)
            n3298 = Select(t=w4372, s=w4371, f=w4374) -> (s? t:f=w4367:string)
            n3299 = case shown="Error" w4352 {
              selector: w4352 -> [w4417 w4463]
              tunnel: [w4415 w4456] -> w4389
              tunnel: w4355 -> [w4418 w4462]
              tunnel: [w4416 w4465] -> w4388
              tunnel: w4386 -> [w4405 w4464]
              tunnel: [w4412 w4464] -> w4387
              frame No Error {
                n3300 = call "Elapsed Time7"() -> ("Time has Elapsed"=w4411:bool)  [unwired: 12 in, 7 out]
                n3301 = Not Equal?(x="Humidity Str Send", y=w4405) -> (x != y?=w4407:bool)
                n3302 = Or(x=w4407, y=w4411) -> (x .or. y?=w4410:bool)
                n3303 = Select(t="Humidity Str Send", s=w4407, f="vals" ("regular expression")) -> (s? t:f=w4406:string)
                n3304 = Or(x=w4410, y="Send") -> (x .or. y?=w4414:bool)
                n3305 = case shown="True" w4414 {
                  tunnel: [w4421 w4426] -> w4415
                  tunnel: w4418 -> [w4420 w4434]
                  tunnel: w4417 -> [w4421 w4433]
                  tunnel: [w4420 w4427] -> w4416
                  tunnel: w4406 -> [_ w4432]
                  tunnel: [w4419 w4423] -> w4412
                  tunnel: "Humidity Str Send" -> [_ w4424]
                  tunnel: w4407 -> [_ w4425]
                  tunnel: w4405 -> [w4419 w4422]
                  frame False {
                  }
                  frame True {
                    n3306 = flat-sequence {
                      tunnel: w4434 -> [w4442]
                      tunnel: w4433 -> [w4441]
                      tunnel: w4432 -> [w4438]
                      tunnel: [w4440] -> w4431
                      tunnel: [w4439] -> w4430
                      tunnel: w4431 -> [w4445]
                      tunnel: w4430 -> [w4444]
                      tunnel: [w4445] -> w4429
                      tunnel: [w4444] -> w4428
                      tunnel: w4429 -> [w4452]
                      tunnel: w4428 -> [w4451]
                      tunnel: [w4450] -> w4427
                      tunnel: [w4449] -> w4426
                      frame #0 {
                        n3307 = local write "Ser Led"(TRUE ("Boolean 4")) -> ()
                        n3308 = Concatenate Strings(w4438, "\r") -> (w4437:string)
                        n3309 = VISA Write(VISA resource name=w4442, write buffer=w4437, error in (no error)=w4441) -> (VISA resource name out=w4440:refnum<visa-resource-name>, error out=w4439:errorcluster)  [unwired: 1 out]
                      }
                      frame #1 {
                        n3310 = Wait (ms)(milliseconds to wait="wait") -> ()  [unwired: 1 out]
                      }
                      frame #2 {
                        w4447 = FALSE ("Send")
                        n3311 = property class="Instr"(reference=w4452, error in=w4451) -> (reference out=w4453:refnum<visa-resource-name>, error out=w4454:errorcluster, "Serial Settings:Number of Bytes at Serial Port"=w4446:u32)
                        n3312 = local write "Send"(w4447) -> ()
                        n3313 = local write "Ser Led"(w4447) -> ()
                        n3314 = VISA Read(VISA resource name=w4453, byte count=w4446, error in (no error)=w4454) -> (VISA resource name out=w4450:refnum<visa-resource-name>, read buffer=→"Humidity Str Rec":string, error out=w4449:errorcluster)  [unwired: 1 out]
                      }
                    }
                    n3315 = Select(t=w4424, s=w4425, f=w4422) -> (s? t:f=w4423:string)
                  }
                }
              }
              frame Error {
                w4470 = u16 0 items=["None"=0, "XON/XOFF"=1, "RTS/CTS"=2, "DTR/DSR"=4] ("flow control")
                w4466 = u16 0 items=["None", "Odd", "Even", "Mark", "Space"] ("parity")
                w4469 = u16 10 items=["1.0"=10, "1.5"=15, "2.0"=20] ("stop bits")
                n3316 = VISA Close(VISA resource name=w4462, error in (no error)=w4463) -> (error out=w4461:errorcluster)
                n3317 = local write "humid"("" ("humid")) -> ()
                n3318 = local write "Humidity Str Rec"("" ("Humidity Str Rec")) -> ()
                n3319 = call <vilib>:"Clear Errors.vi"("error in (no error)"=w4461) -> ("error out"=w4460:errorcluster)  [unwired: 5 in, 1 out]
                n3320 = local read "Com Port 3"() -> (w4459:refnum<visa-resource-name>)
                n3321 = call-poly "VISA Configure Serial Port"("VISA resource name"=w4459, "timeout (10sec)"=u32 1000, "termination char\n(0xA = '\\n' = LF)"=u8 10 ("termination char\n(0xA = '\\n' = LF)"), "Enable Termination\nChar (T)"=FALSE ("Enable Termination Char (T)"), "data bits (8)"=u16 8 ("data bits"), "parity (0:none)"=w4466, "error in (no error)"=w4460, "stop bits (10: 1 bit)"=w4469, "flow control (0:none)"=w4470) -> ("VISA resource name out"=w4465:refnum<visa-resource-name>, "baud rate (9600)"=w4457:u32, "error out"=w4456:errorcluster)  [unwired: 4 in]
              }
            }
            n3322 = Compound Arithmetic op=AND(w4361, w4360, w4362) -> (w4359:bool)
            n3323 = case shown="True" w4359 {
              tunnel: w4358 -> [_ _]
              tunnel: w4367 -> [_ w4397]
              frame False {
              }
              frame True {
                w4395 = " " ("regular expression")
                n3324 = Match Pattern(string=w4397, regular expression=" ") -> (after substring=w4399:string)  [unwired: 1 in, 3 out]
                n3325 = Match Pattern(string=w4399, regular expression=w4395) -> (before substring=→"humid":string, after substring=w4396:string)  [unwired: 1 in, 2 out]
                n3326 = Match Pattern(string=w4396, regular expression=w4395) -> (before substring=→"temp_@Rh sensor":string)  [unwired: 1 in, 3 out]
              }
            }
            n3327 = local read "Quit"() -> (w4348:bool)
          }
          n3328 = VISA Close(VISA resource name=w4344, error in (no error)=w4345) -> (error out=w4341:errorcluster)
          n3329 = call <vilib>:"Clear Errors.vi"("error in (no error)"=w4341) -> ()  [unwired: 5 in, 2 out]
        }
        frame Enabled {
        }
      }
    }
    frame Enabled {
    }
  }
  n3330 = while {
    tunnel: [w4477] -> _
    i -> [w4477]
    stop <- w4473 stop-if-true
    # "Langauage selection"
    n3331 = Equal?(x="Lan flag", y=22.0) -> ()  [unwired: 1 out]
    n3332 = disable-structure shown="Disabled" {
      frame Disabled {
        n3333 = stacked-sequence {
          frame #0 {
            n3334 = case shown="\"Russian\"" "Language Selection" {
              tunnel: [0 1] -> w4479
              frame "English", Default {
              }
              frame "Russian" {
              }
            }
            n3335 = for {
              N: 130 -> [_]
              tunnel: "Table" -> [w4488]
              tunnel: w4479 -> [w4487]
              i -> [w4486]
              n3336 = Index Array(array=w4488, index (row)=w4486, index (col)=w4487) -> (element=w4485:string)
              n3337 = case shown="123" w4486 {
                tunnel: w4485 -> [w4489 w4490 _ w4491 w4492 w4493 w4494 w4495 w4496 w4497 w4498 w4499 w4500 w4501 w4502 w4503 w4504 w4505 w4506 w4507 w4508 w4509 w4510 w4511 w4512 w4513 w4514 w4515 w4516 _ _ w4517 w4518 w4519 w4520 w4521 w4522 w4531 w4538 w4545 w4552 w4556 w4559 w4562 w4564 w4566 w4567 w4568 w4569 w4570 w4571 w4572 w4573 w4574 w4575 w4576 w4577 w4578 w4579 w4580 w4581 w4582 w4583 w4584 w4585 w4586 w4587 w4588 w4589 w4590 w4591 w4592 w4593 w4594 w4595 w4596 w4597 w4598 w4599 w4600 w4601 w4602 w4603 w4604 w4605 w4606 w4607 w4608 w4609 w4610 w4611 w4612 w4613 w4614 w4615 w4616 w4617 w4618 w4619 w4620 w4621 w4622 w4623 w4624 w4625 _ w4626 w4627 w4628 w4629 w4630 w4631 w4632 w4633 w4634 w4635 w4636 w4637 w4638 _ w4639 w4640 w4641 w4642 w4643 w4644 _]
                frame 0 {
                  n3338 = local write "S"(w4489) -> ()
                }
                frame 1 {
                  n3339 = local write "S 2"(w4490) -> ()
                }
                frame 2 {
                }
                frame 3 {
                  n3340 = local write "S 4"(w4491) -> ()
                }
                frame 4 {
                  n3341 = property on="FILE" class="Str"("Caption.Text"=w4492) -> ()  [unwired: 2 in, 2 out]
                }
                frame 5 {
                  n3342 = property on="Fuel Discription :" class="Str"("Caption.Text"=w4493) -> ()  [unwired: 2 in, 2 out]
                }
                frame 6 {
                  n3343 = property on="Remarks :" class="Str"("Caption.Text"=w4494) -> ()  [unwired: 2 in, 2 out]
                }
                frame 7 {
                  n3344 = property on="Save & Continue" class="Bool (strict)"("Boolean Text.Text"=w4495) -> ()  [unwired: 2 in, 2 out]
                }
                frame 8 {
                }
                frame 9 {
                  n3345 = property on="Set Hz" class="DigNum (strict)"("Caption.Text"=w4497) -> ()  [unwired: 2 in, 2 out]
                }
                frame 10 {
                  "String 3" <- w4498
                }
                frame 11 {
                  n3346 = property on="NORMAL LOAD" class="DigNum (strict)"("Caption.Text"=w4499) -> ()  [unwired: 2 in, 2 out]
                }
                frame 12 {
                  "String 5" <- w4500
                }
                frame 13 {
                  n3347 = property on="Set Temp" class="DigNum (strict)"("Caption.Text"=w4501) -> ()  [unwired: 2 in, 2 out]
                }
                frame 14 {
                  n3348 = local write "S 15"(w4502) -> ()
                }
                frame 15 {
                  n3349 = property on="Set Rh" class="DigNum (strict)"("Caption.Text"=w4503) -> ()  [unwired: 2 in, 2 out]
                }
                frame 16 {
                  "String 13" <- w4504
                  "String 26" <- w4504
                }
                frame 17 {
                  n3350 = local write "S 18"(w4505) -> ()
                }
                frame 18 {
                  "String 17" <- w4506
                }
                frame 19 {
                  n3351 = property on="test time" class="DigNum (strict)"("Caption.Text"=w4507) -> ()  [unwired: 2 in, 2 out]
                }
                frame 20 {
                  "String 18" <- w4508
                  "String 22" <- w4508
                }
                frame 21 {
                  n3352 = property on="Elapsed time" class="DigNum (strict)"("Caption.Text"=w4509) -> ()  [unwired: 2 in, 2 out]
                }
                frame 22 {
                  n3353 = property on="Samplingtime 2" class="DigNum (strict)"("Caption.Text"=w4510) -> ()  [unwired: 2 in, 2 out]
                }
                frame 23 {
                  "String 21" <- w4511
                }
                frame 24 {
                  n3354 = property on="Countdown" class="DigNum (strict)"("Caption.Text"=w4512) -> ()  [unwired: 2 in, 2 out]
                }
                frame 25 {
                  n3355 = property on="Countdown 2" class="DigNum (strict)"("Caption.Text"=w4513) -> ()  [unwired: 2 in, 2 out]
                }
                frame 26 {
                  n3356 = property on="Engage" class="Bool (strict)"("Boolean Text.Text"=w4514) -> ()  [unwired: 2 in, 2 out]
                }
                frame 27 {
                  n3357 = property on="Boolean  4" class="Bool (strict)"("Boolean Text.Text"=w4515) -> ()  [unwired: 2 in, 2 out]
                }
                frame 28 {
                  n3358 = property on="Test \nStatus" class="Bool (strict)"("Boolean Text.Text"=w4516) -> ()  [unwired: 2 in, 2 out]
                }
                frame 29 {
                }
                frame 30 {
                }
                frame 31 {
                }
                frame 32 {
                  n3359 = property on="RSTCOF" class="Bool"("Boolean Text.Text"=w4518) -> ()  [unwired: 2 in, 2 out]
                  n3360 = property on="RST FF" class="Bool"("Boolean Text.Text"=w4518) -> ()  [unwired: 2 in, 2 out]
                  n3361 = property on="RST TEMP" class="Bool"("Boolean Text.Text"=w4518) -> ()  [unwired: 2 in, 2 out]
                  n3362 = property on="RSTV1 3" class="Bool"("Boolean Text.Text"=w4518) -> ()  [unwired: 2 in, 2 out]
                  n3363 = property on="rstv2" class="Bool"("Boolean Text.Text"=w4518) -> ()  [unwired: 2 in, 2 out]
                  n3364 = property on="RSTV1 2" class="Bool"("Boolean Text.Text"=w4518) -> ()  [unwired: 2 in, 2 out]
                  n3365 = property on="RST CP" class="Bool"("Boolean Text.Text"=w4518) -> ()  [unwired: 2 in, 2 out]
                }
                frame 33 {
                  "S 61" <- w4519
                }
                frame 34 {
                  "String 23" <- w4520
                }
                frame 35 {
                  n3366 = property on="Rh Before" class="DigNum (strict)"("Caption.Text"=w4521) -> ()  [unwired: 2 in, 2 out]
                }
                frame 36 {
                  n3367 = Match Pattern(string=w4522, regular expression=",") -> (before substring=→"bs":string, after substring=→"as":string)  [unwired: 1 in, 2 out]
                  n3368 = property on="Rh After" class="DigNum (strict)"("Caption.Text"=w4522) -> ()  [unwired: 2 in, 2 out]
                }
                frame 37 {
                  n3369 = Match Pattern(string=w4531, regular expression=",") -> (before substring=w4530:string, after substring=w4529:string)  [unwired: 1 in, 2 out]
                  "bs" <- w4530
                  "as" <- w4529
                  n3370 = Concatenate Strings(w4530, w4529) -> (w4526:string)
                  n3371 = property on="Humidity before test 2" class="DigNum (strict)"("Caption.Text"=w4526) -> ()  [unwired: 2 in, 2 out]
                  n3372 = property on="Humidity before test" class="DigNum (strict)"("Caption.Text"=w4526) -> ()  [unwired: 2 in, 2 out]
                  n3373 = Concatenate Strings(w4526, "=" ("string")) -> (w4527:string)
                  n3374 = local write "S 38"(w4527) -> ()
                }
                frame 38 {
                  n3375 = Match Pattern(string=w4538, regular expression=",") -> (before substring=w4537:string, after substring=w4536:string)  [unwired: 1 in, 2 out]
                  "bs" <- w4537
                  "as" <- w4536
                  n3376 = Concatenate Strings(w4537, w4536) -> (w4533:string)
                  n3377 = property on="Humidity after test 2" class="DigNum (strict)"("Caption.Text"=w4533) -> ()  [unwired: 2 in, 2 out]
                  n3378 = Concatenate Strings(w4533, "=" ("string")) -> (w4535:string)
                  n3379 = property on="Humidity after test" class="DigNum (strict)"("Caption.Text"=w4533) -> ()  [unwired: 2 in, 2 out]
                  n3380 = local write "S 39"(w4535) -> ()
                }
                frame 39 {
                  n3381 = Match Pattern(string=w4545, regular expression=",") -> (before substring=w4544:string, after substring=w4543:string)  [unwired: 1 in, 2 out]
                  "bs" <- w4544
                  "as" <- w4543
                  n3382 = Concatenate Strings(w4544, w4543) -> (w4540:string)
                  n3383 = property on="Temperature before test 2" class="DigNum (strict)"("Caption.Text"=w4540) -> ()  [unwired: 2 in, 2 out]
                  n3384 = property on="Temperature before test" class="DigNum (strict)"("Caption.Text"=w4540) -> ()  [unwired: 2 in, 2 out]
                  n3385 = Concatenate Strings(w4540, "=" ("string")) -> (→"String 34":string)
                }
                frame 40 {
                  n3386 = Match Pattern(string=w4552, regular expression=",") -> (before substring=w4551:string, after substring=w4550:string)  [unwired: 1 in, 2 out]
                  "bs" <- w4551
                  "as" <- w4550
                  n3387 = Concatenate Strings(w4551, w4550) -> (w4547:string)
                  n3388 = property on="Temperature after test 2" class="DigNum (strict)"("Caption.Text"=w4547) -> ()  [unwired: 2 in, 2 out]
                  n3389 = Concatenate Strings(w4547, "=" ("string")) -> (→"String 35":string)
                  n3390 = property on="Temperature after test" class="DigNum (strict)"("Caption.Text"=w4547) -> ()  [unwired: 2 in, 2 out]
                }
                frame 41 {
                  n3391 = property on="AVP" class="DigNum (strict)"("Caption.Text"=w4556) -> ()  [unwired: 2 in, 2 out]
                  n3392 = property on="AVP 2" class="DigNum (strict)"("Caption.Text"=w4556) -> ()  [unwired: 2 in, 2 out]
                  n3393 = Concatenate Strings(w4556, "=" ("string")) -> (→"String 36":string)
                }
                frame 42 {
                  n3394 = property on="MWSD" class="DigNum (strict)"("Caption.Text"=w4559) -> ()  [unwired: 2 in, 2 out]
                  n3395 = property on="MWSD 2" class="DigNum (strict)"("Caption.Text"=w4559) -> ()  [unwired: 2 in, 2 out]
                  n3396 = Concatenate Strings(w4559, "=" ("string")) -> (→"String 37":string)
                }
                frame 43 {
                  n3397 = property on="HCF 2" class="DigNum (strict)"("Caption.Text"=w4562) -> ()  [unwired: 2 in, 2 out]
                  n3398 = property on="HCF" class="DigNum (strict)"("Caption.Text"=w4562) -> ()  [unwired: 2 in, 2 out]
                  n3399 = Concatenate Strings(w4562, "=" ("string")) -> (→"String 38":string)
                }
                frame 44 {
